vi "Flock_LocalProcessTemplate_Process.vi"(11 "Process":string) -> ()   [LabVIEW 2014]
uses:
  LocalProcessMessaging/Flock_Shared_LocalProcessMessaging.lvlib
  CentralProcessMessaging/Flock_Shared_CentralProcessMessaging.lvlib
  Error Handling/Flock_ErrorHandling.lvlib
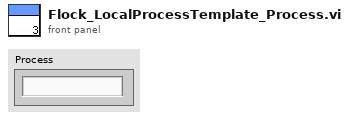
[diagram p1: front panel]
types:
  T1 = typedef "Flock_Shared_Messaging.lvlib/ProcessList.ctl" = string
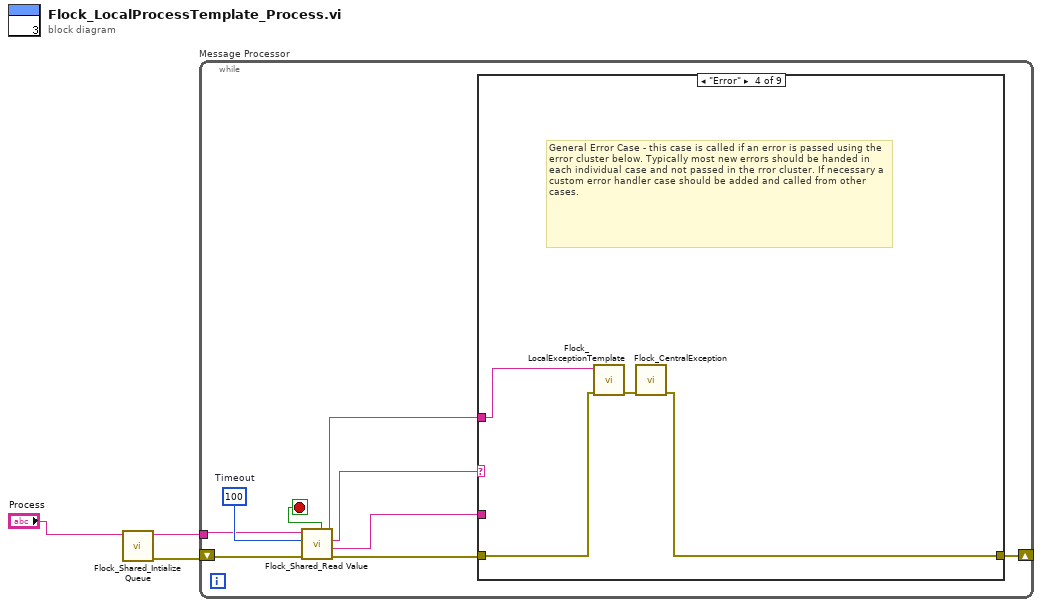
[diagram p0: block diagram]
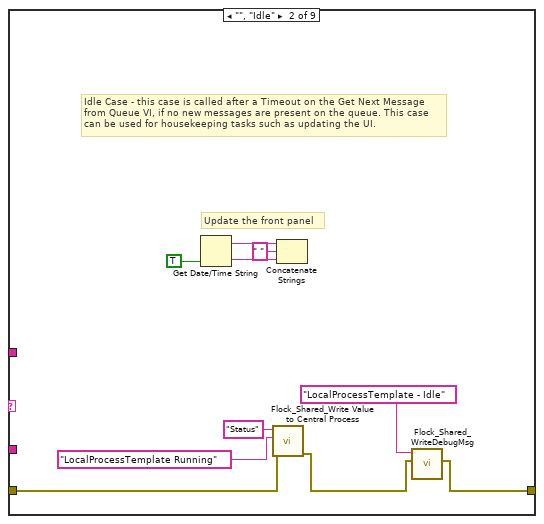
[diagram p3: hidden frame]
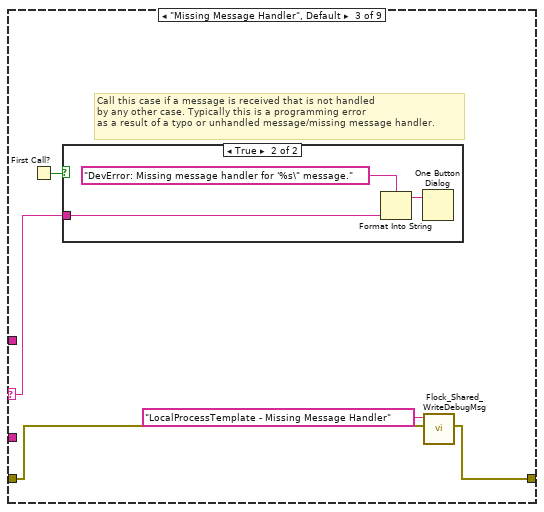
[diagram p4: hidden frame]
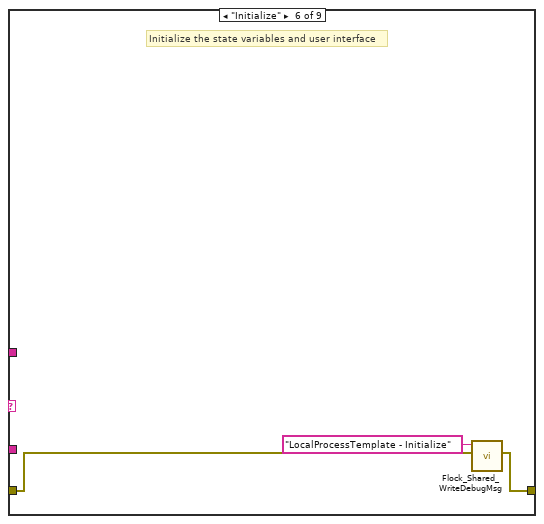
[diagram p7: hidden frame]
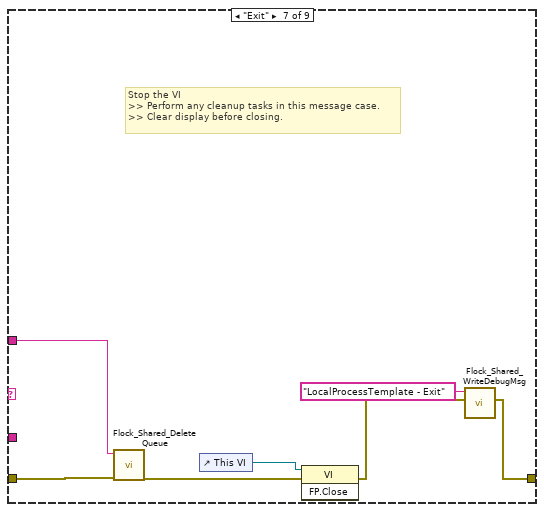
[diagram p8: hidden frame]
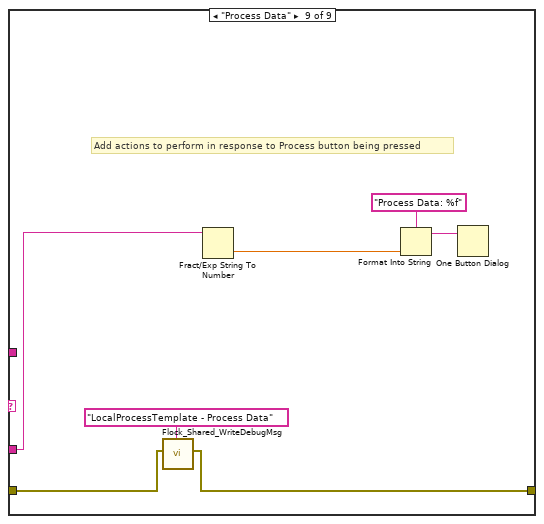
[diagram p10: hidden frame]
diagram:
  n1 = call "Flock_Shared_Intialize Queue.vi"("Enum"="Process") -> ("error out"=w2:errorcluster, "Process Name"=w1:T1)  [unwired: 9 in]
  n2 = while "Message Processor" {
    shift-left: w2 -> [w10]
    shift-right: [w12] -> _
    tunnel: w1 -> [w5]
    stop <- w6 stop-if-true
    w11 = 100  # Timeout
    n3 = call "Flock_Shared_Read Value.vi"("error in (no error)"=w10, "timeout (1ms)"=w11, "Process"=w5) -> ("error out"=w9:errorcluster, "Message Value"=w7:string, "Message Name"=w8:string, "Process"=w4:T1, "Exit Process"=w6:bool)  [unwired: 4 in]
    n4 = case shown="\"Error\"" w8 {
      selector: w8 -> [_ _ w28 _ _ _ _ _ _]
      tunnel: [w13 w15 w26 w34 w36 w38 w41 w47 w49] -> w12
      tunnel: w9 -> [w13 w17 w27 w33 w36 w39 w46 w47 w50]
      tunnel: w7 -> [_ _ _ _ _ _ _ _ w51]
      tunnel: w4 -> [_ _ _ w32 _ _ w45 _ _]
      frame "---------- Framework Operations ----------" {
        # "Dummy case to add a seperator in the Case Structure menu"
      }
      frame "", "Idle" {
        # "Update the front panel"
        # "Idle Case - this case is called after a Timeout on the Get Next Message from Queue VI, if no new messages are present on the queue. This case can be used for housekeeping tasks such as updating the UI."
        n5 = Get Date/Time String(want seconds? (F)=TRUE) -> (date string=w23:string, time string=w22:string)  [unwired: 2 out]
        n6 = call "Flock_Shared_Write Value to Central Process.vi"("error in (no error)"=w17, "Message Value"="LocalProcessTemplate Running", "Message Name"="Status") -> ("error out"=w16:errorcluster)  [unwired: 8 in]
        n7 = Concatenate Strings(w23, " " ("string"), w22) -> ()  [unwired: 1 out]
        n8 = call "Flock_Shared_WriteDebugMsg.vi"("error in (no error)"=w16, "Current Message Case"="LocalProcessTemplate - Idle") -> ("error out"=w15:errorcluster)  [unwired: 9 in]
      }
      frame "Missing Message Handler", Default {
        # "Call this case if a message is received that is not handled \nby any other case. Typically this is a programming error\nas a result of a typo or unhandled message/missing message handler."
        n9 = First Call?() -> (First Call?: T/F=w24:bool)
        n10 = case shown="True" w24 {
          tunnel: w28 -> [_ w31]
          frame False {
          }
          frame True {
            n11 = Format Into String(format string="DevError: Missing message handler for '%s\" message." ("message"), w31) -> (resulting string=w29:string)  [unwired: 2 in, 1 out]
            n12 = One Button Dialog(message=w29) -> ()  [unwired: 2 out]
          }
        }
        n13 = call "Flock_Shared_WriteDebugMsg.vi"("error in (no error)"=w27, "Current Message Case"="LocalProcessTemplate - Missing Message Handler") -> ("error out"=w26:errorcluster)  [unwired: 9 in]
      }
      frame "Error" {
        # "General Error Case - this case is called if an error is passed using the error cluster below. Typically most new errors should be handed in each individual case and not passed in the rror cluster. If necessary a custom error handler case should be added and called from other cases."
        n14 = call "Flock_LocalExceptionTemplate.vi"("Error In"=w33, "Process List"=w32) -> ("Error Out"=w35:errorcluster)  [unwired: 9 in]
        n15 = call "Flock_CentralException.vi"("Error In"=w35) -> ("Error Out"=w34:errorcluster)  [unwired: 10 in]
      }
      frame "---------- Generic Operations ----------" {
        # "Dummy case to add a seperator in the Case Structure menu"
      }
      frame "Initialize" {
        # "Initialize the state variables and user interface"
        n16 = call "Flock_Shared_WriteDebugMsg.vi"("error in (no error)"=w39, "Current Message Case"="LocalProcessTemplate - Initialize") -> ("error out"=w38:errorcluster)  [unwired: 9 in]
      }
      frame "Exit" {
        # "Stop the VI\n>> Perform any cleanup tasks in this message case.\n>> Clear display before closing."
        n17 = call "Flock_Shared_Delete Queue.vi"("Error In"=w46, "Process Name"=w45) -> ("Error Out"=w43:errorcluster)  [unwired: 9 in]
        n18 = control-ref of="This VI"() -> (w44:refnum<vi>)
        n19 = invoke class="VI" method="FP.Close"(reference=w44, error in=w43) -> (error out=w42:errorcluster)  [unwired: 1 in, 2 out]
        n20 = call "Flock_Shared_WriteDebugMsg.vi"("error in (no error)"=w42, "Current Message Case"="LocalProcessTemplate - Exit") -> ("error out"=w41:errorcluster)  [unwired: 9 in]
      }
      frame "---------- Application Operations ----------" {
        # "Dummy case to add a seperator in the Case Structure menu"
      }
      frame "Process Data" {
        # "Add actions to perform in response to Process button being pressed"
        n21 = call "Flock_Shared_WriteDebugMsg.vi"("error in (no error)"=w50, "Current Message Case"="LocalProcessTemplate - Process Data") -> ("error out"=w49:errorcluster)  [unwired: 9 in]
        n22 = Fract/Exp String To Number(string=w51) -> (number=w54:dbl)  [unwired: 4 out]
        n23 = Format Into String(format string="Process Data: %f" ("message"), w54) -> (resulting string=w52:string)  [unwired: 2 in, 1 out]
        n24 = One Button Dialog(message=w52) -> ()  [unwired: 2 out]
      }
    }
  }
